vi "create.DeleteOrder.vi"(8 "error in":errorcluster, 10 "DeleteOrder.Parameters":T1, 11 "DeleteOrder in":refnum<class "DeleteOrder.lvclass">) -> (0 "error out":errorcluster, 3 "DeleteOrder out":refnum<class "DeleteOrder.lvclass">)   [LabVIEW 2020, in "DeleteOrder.lvclass"]
uses:
  DeleteOrder.lvclass
  DeleteOrder.Parameters.ctl
  FieldSpec.ctl
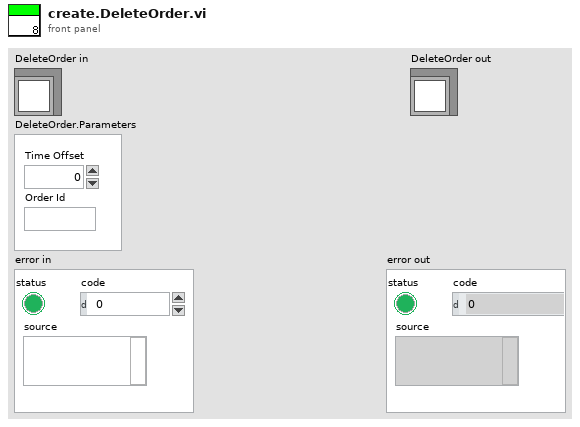
[diagram p1: front panel]
types:
  T1 = typedef "DeleteOrder.lvclass/DeleteOrder.Parameters.ctl" = cluster{"Time Offset":u32, "Order Id":string}
  T2 = typedef "FieldSpec.ctl" = cluster{"Name":string, "Offset":i32, "Length":i32, "FieldType":enum16{"Alphanumeric", "Binary", "BinaryLongPrice", "BinaryShortPrice", "BitField", "PrintableAscii", "Value"}, "FieldValue":variant}
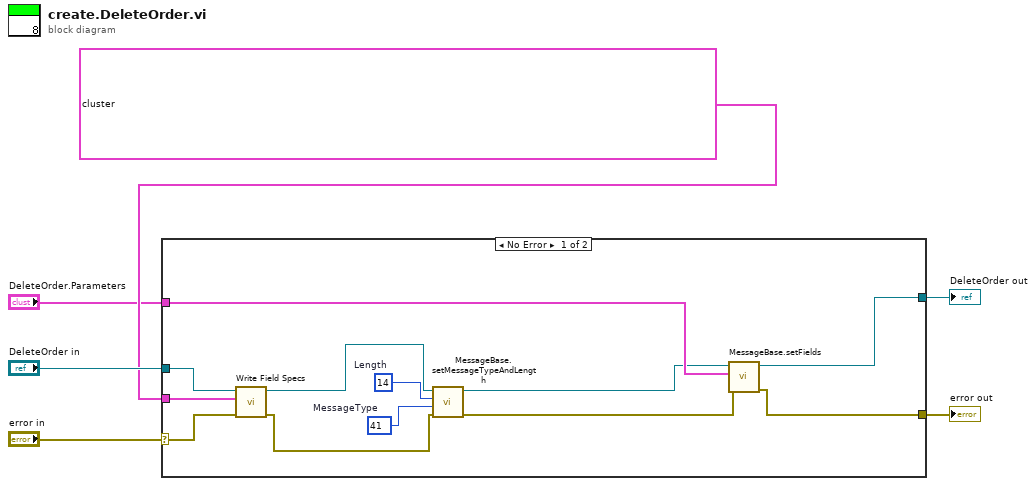
[diagram p0: block diagram]
diagram:
  n1 = case shown="No Error" "error in" {
    selector: "error in" -> [w16 w20]
    tunnel: [w8 w20] -> w5
    tunnel: [w7 w19] -> w3
    tunnel: "DeleteOrder in" -> [w18 w19]
    tunnel: T2[] [{"Name"="Length", "Offset"=0, "Length"=1, "FieldType"=enum."Binary", "FieldValue"=variant}, {"Name"="MessageType", "Offset"=1, "Length"=1, "FieldType"=enum."Value", "FieldValue"=variant}, {"Name"="Time Offset", "Offset"=2, "Length"=4, "FieldType"=enum."Binary", "FieldValue"=variant}, {"Name"="Order Id", "Offset"=6, "Length"=8, "FieldType"=enum."Binary", "FieldValue"=variant}] ("appended array") -> [w17 _]
    tunnel: "DeleteOrder.Parameters" -> [w11 _]
    frame No Error {
      w15 = u8 41  # MessageType
      w14 = u8 14  # Length
      n2 = call-dynamic "Write Field Specs.vi"("error in (no error)"=w16, "Field Specs"=w17, "MessageBase in"=w18) -> ("error out"=w13:errorcluster, "MessageBase out"=w12:refnum<class "DeleteOrder.lvclass">)  [unwired: 7 in]
      n3 = call-dynamic "MessageBase.setMessageTypeAndLength.vi"("error in (no error)"=w13, "MessageType"=w15, "Length"=w14, "MessageBase in"=w12) -> ("error out"=w9:errorcluster, "MessageBase out"=w10:refnum<class "DeleteOrder.lvclass">)  [unwired: 6 in]
      n4 = call-dynamic "MessageBase.setFields.vi"("error in (no error)"=w9, "Cluster (dup)"=w11, "MessageBase in"=w10) -> ("error out"=w8:errorcluster, "MessageBase out"=w7:refnum<class "DeleteOrder.lvclass">)  [unwired: 7 in]
    }
    frame Error {
    }
  }
  "error out" <- w5
  "DeleteOrder out" <- w3
